vi "WS1050 36 DUT CV Curve Ver1.3.vi"() -> ()   [LabVIEW 2012]
uses:
  WS_VCAP Driver 029/Source/WSVCAP Shell/Type Defs/WSVCAP SHL I2C DUT Mask Mode Enum.ctl
panel:
  out "date string":string="5/19/2014"
  in  "Tab Control":T1(tab)
  in  "Sweep CP":bool=TRUE
  in  "Board#":string="BRD5"
  in  "Serial Number":string[][](table)=[["DUT", "SN"], ["DUT1", "1"], ["DUT2", "2"], ["DUT3", "3"], ["DUT4", "4"], ["DUT5", "5"], ["DUT6", "6"], ["DUT7", "7"], ["DUT8", "8"], ["DUT9", "9"], ["DUT10", "10"], ["DUT11", "11"], ["DUT12", "12"], ["DUT13", "13"], ["DUT14", "14"], ["DUT15", "15"], ["DUT16", "16"], ["DUT17", "17"], ["DUT18", "18"], ["DUT19", "19"], ["DUT20", "20"], ["DUT21", "21"], ["DUT22", "22"], ["DUT23", "23"], ["DUT24", "24"], ["DUT25", "25"], ["DUT26", "26"], ["DUT27", "27"], ["DUT28", "28"], ["DUT29", "29"], ["DUT30", "30"], ["DUT31", "31"], ["DUT32", "32"], ["DUT33", "33"], ["DUT34", "34"], ["DUT35", "35"], ["DUT36", "36"]]
  in  "Wafer#":string="T7-EB"
  in  "File Name":string="CP Sweep_WS1050_T7_EB_25C_BRD4_160706_1"
  in  "TMN DC\\CAP Data Log File Path":path=path "C:/WS1050 36 DUT Data"
  in  "Test Program":string="WS1050 36 DUT CV Curve Ver1.3"
  out "Current Date":string="8/28/2014"
  out "Current Time":string="0950"
  in  "Start Date":string="10/21/2014"
  in  "Start Time":string="1542"
  in  "Comment":string="CP Sweep RT"
  in  "OK Button":bool
  in  "Calibration":bool
  in  "Verify CP":bool
  in  "CP Setting":i32(ring) items=["CP OFF", "CP ON", "CP 35V", "CP 40V", "DVA ON", "DVA OFF", "REG1 ON", "REG1 OFF", "REG2 ON", "REG2 OFF", "REG3 ON", "REG3 OFF"]
  in  "Set VDD":dbl=3.3 format="%.3g"
  in  "Clock Rate (Hz)":dbl=1000000.0 caption="Meas Speed" format="%.1p Hz"
  out "AR  Measurent(Hz)":dbl
  in  "PS1 Source":refnum<visa-resource-name>="GPIB0::5::INSTR"
  in  "Ke2000":refnum<visa-resource-name>="GPIB0::9::INSTR"
  out "Simulate FPGA":bool
  out "Online":bool
  in  "Ke2400":refnum<visa-resource-name>="GPIB0::3::INSTR"
  in  "Initialize AD7747":bool
  in  "DUT Mask Mode":T2=enum."All"
  in  "RFFE Slave Address":u8=7 caption="Slave Address" format="0x%02x"
  out "Activity Log":string="05/19/2014 -- 12:24:35.853::WSVCAP::APP::Application Started\n05/19/2014 -- 12:24:37.606::WSVCAP::WSVCAP SHL::WR I2C-REG:0x0A;MASK:0xFFFFFFFFFFFF;C1 DATA:22:22:22:22:22:22:22:22:22:22:22:22:22:22:22:22;C2 DATA:22:22:22:22:22:22:22:22:22:22:22:22:22:22:22:22;C3 DATA:22:22:22:22:22:22:22:22:22:22:22:22:22:22:22:22\r\n05/19/2014 -- 12:24:37.773::WSVCAP::WSVCAP SHL::WR I2C-ST:0,0,4,1\r\n05/19/2014 -- 12:24:37.903::WSVCAP::WSVCAP SHL::RD I2C-BYTES:4;ADD:0x00;MASK:0xFFFFFFFFFFFF\r\n05/19/2014 -- 12:24:38.045::WSVCAP::WSVCAP SHL::RD I2C:C1 DATA:2:2:2:2:2:2:2:2:2:2:2:2:2:2:2:2|A7:A9:AA:82:82:7F:82:81:82:81:83:82:81:82:82:81|46:36:BB:88:44:A3:E9:2B:32:20:ED:25:BB:3D:68:B|2C:6A:EB:A7:22:56:FE:CC:36:82:D7:B0:3B:48:F9:CC;C2 DATA:2:2:2:2:2:2:2:2:2:2:2:2:2:2:2:2|94:94:94:80:80:80:80:80:81:7E:7E:81:80:7E:80:80|47:33:15:82:62:B:E8:1C:D7:C3:7D:41:7C:B7:4C:2A|C4:B4:AE:8:1E:D1:4E:37:11:C0:6F:63:42:9D:63:B5;C3 DATA:2:2:2:2:2:2:2:2:2:2:2:2:2:2:2:2|95:95:95:81:81:7E:81:80:84:7D:80:83:81:7E:7F:80|AB:C4:14:B5:7B:52:DF:C9:79:5D:5F:30:99:31:1E:F4|6E:5C:F7:A8:C3:EB:7B:EF:33:92:89:77:4D:67:75:DD;STATUS:0:0:4:0\r\n05/19/2014 -- 12:24:38.046::WSVCAP::WSVCAP SHL::WR I2C-REG:0x0A;MASK:0xFFFFFFFFFFFF;C1 DATA:22:22:22:22:22:22:22:22:22:22:22:22:22:22:22:22;C2 DATA:22:22:22:22:22:22:22:22:22:22:22:22:22:22:22:22;C3 DATA:22:22:22:22:22:22:22:22:22:22:22:22:22:22:22:22\r\n05/19/2014 -- 12:24:38.089::WSVCAP::WSVCAP SHL::WR I2C-ST:0,0,4,1\r\n05/19/2014 -- 12:24:38.219::WSVCAP::WSVCAP SHL::RD I2C-BYTES:4;ADD:0x00;MASK:0xFFFFFFFFFFFF\r\n05/19/2014 -- 12:24:38.362::WSVCAP::WSVCAP SHL::RD I2C:C1 DATA:2:2:2:2:2:2:2:2:2:2:2:2:2:2:2:2|A7:AB:AA:82:82:82:83:83:82:82:82:82:7F:82:82:81|4B:32:96:83:3E:61:43:17:25:62:AB:4D:A2:40:2E:5|3C:76:2B:B4:EE:E4:A9:1A:AA:A:26:C7:21:2E:87:5B;C2 DATA:2:2:2:2:2:2:2:2:2:2:2:2:2:2:2:2|94:94:94:80:80:80:80:80:80:7F:80:81:80:80:7F:80|4A:32:19:7D:19:6C:79:46:61:7F:4B:B8:A5:30:F3:14|B4:70:A:8C:9C:DC:43:FA:1E:A:C6:21:A:A9:13:F3;C3 DATA:2:2:2:2:2:2:2:2:2:2:2:2:2:2:2:2|95:97:94:81:80:81:82:81:80:7E:81:84:7F:81:80:80|B2:32:D0:A7:9E:4C:AB:D4:EE:D9:F0:82:B7:91:7:FF|C1:91:B6:3D:D8:E:1B:4F:9F:6A:F1:6C:E7:3F:7:BA;STATUS:0:0:4:0\r\n05/19/2014 -- 12:24:38.364::WSVCAP::WSVCAP SHL::WR I2C-REG:0x0A;MASK:0xFFFFFFFFFFFF;C1 DATA:22:22:22:22:22:22:22:22:22:22:22:22:22:22:22:22;C2 DATA:22:22:22:22:22:22:22:22:22:22:22:22:22:22:22:22;C3 DATA:22:22:22:22:22:22:22:22:22:22:22:22:22:22:22:22\r\n05/19/2014 -- 12:24:38.406::WSVCAP::WSVCAP SHL::WR I2C-ST:0,0,4,1\r\n05/19/2014 -- 12:24:38.536::WSVCAP::WSVCAP SHL::RD I2C-BYTES:4;ADD:0x00;MASK:0xFFFFFFFFFFFF\r\n05/19/2014 -- 12:24:38.678::WSVCAP::WSVCAP SHL::RD I2C:C1 DATA:2:2:2:2:2:2:2:2:2:2:2:2:2:2:2:2|A7:A9:AB:82:82:81:82:82:82:82:82:82:82:82:82:81|46:71:4C:87:43:3D:7F:FC:25:4F:8E:54:97:3E:60:8C|AA:F4:1F:B5:CE:43:1F:36:9:87:9C:78:86:5:B6:8E;C2 DATA:2:2:2:2:2:2:2:2:2:2:2:2:2:2:2:2|94:94:94:80:7F:7F:80:80:80:80:80:81:80:80:80:80|49:36:18:7D:6E:C5:E4:3C:81:2E:41:D3:75:71:E3:72|E8:D3:E6:D1:E0:48:AE:D4:54:D:E8:8E:B4:41:68:4;C3 DATA:2:2:2:2:2:2:2:2:2:2:2:2:2:2:2:2|95:95:95:81:7F:7F:81:81:81:81:81:84:81:81:82:81|B3:F5:90:AB:82:69:7B:93:D0:77:E8:D5:E8:8C:84:E8|B9:AC:EE:2B:B6:71:8F:4A:74:31:56:BB:8A:B7:A0:C8;STATUS:0:0:4:0\r\n05/19/2014 -- 12:24:38.681::WSVCAP::WSVCAP SHL::WR I2C-REG:0x0A;MASK:0xFFFFFFFFFFFF;C1 DATA:22:22:22:22:22:22:22:22:22:22:22:22:22:22:22:22;C2 DATA:22:22:22:22:22:22:22:22:22:22:22:22:22:22:22:22;C3 DATA:22:22:22:22:22:22:22:22:22:22:22:22:22:22:22:22\r\n05/19/2014 -- 12:24:38.723::WSVCAP::WSVCAP SHL::WR I2C-ST:0,0,4,1\r\n05/19/2014 -- 12:24:38.854::WSVCAP::WSVCAP SHL::RD I2C-BYTES:4;ADD:0x00;MASK:0xFFFFFFFFFFFF\r\n05/19/2014 -- 12:24:38.996::WSVCAP::WSVCAP SHL::RD I2C:C1 DATA:2:2:2:2:2:2:2:2:2:2:2:2:2:2:2:2|A7:A9:AA:82:82:7F:83:81:82:81:84:82:7F:82:7F:82|43:FB:E:7F:3C:AD:35:35:26:A2:6C:21:4B:3D:8:6|63:9A:E1:F3:95:32:91:42:90:3C:78:1F:5C:D7:5F:D8;C2 DATA:2:2:2:2:2:2:2:2:2:2:2:2:2:2:2:2|94:94:94:80:80:80:80:80:81:80:7E:81:80:7E:7F:80|48:36:18:7F:5E:3D:69:83:DE:AE:A1:9E:31:AE:BB:96|15:A0:44:17:13:FD:CC:C8:6D:B2:EF:A7:C:C7:3B:F;C3 DATA:2:2:2:2:2:2:2:2:2:2:2:2:2:2:2:2|95:96:94:81:81:7E:82:80:84:80:80:84:7F:7E:7D:82|AD:3B:6D:A9:7C:57:9D:F5:7A:96:23:5C:36:2D:ED:5A|CD:46:DB:3B:C7:BD:70:60:33:B8:B:F7:63:A:51:4D;STATUS:0:0:4:0\r\n05/19/2014 -- 12:24:38.998::WSVCAP::WSVCAP SHL::WR I2C-REG:0x0A;MASK:0xFFFFFFFFFFFF;C1 DATA:22:22:22:22:22:22:22:22:22:22:22:22:22:22:22:22;C2 DATA:22:22:22:22:22:22:22:22:22:22:22:22:22:22:22:22;C3 DATA:22:22:22:22:22:22:22:22:22:22:22:22:22:22:22:22\r\n05/19/2014 -- 12:24:39.040::WSVCAP::WSVCAP SHL::WR I2C-ST:0,0,4,1\r\n05/19/2014 -- 12:24:39.170::WSVCAP::WSVCAP SHL::RD I2C-BYTES:4;ADD:0x00;MASK:0xFFFFFFFFFFFF\r\n05/19/2014 -- 12:24:39.311::WSVCAP::WSVCAP SHL::RD I2C:C1 DATA:2:2:2:2:2:2:2:2:2:2:2:2:2:2:2:2|A7:AA:AB:82:82:81:82:81:82:81:82:82:82:82:7F:82|44:F1:90:87:45:44:C8:2C:2C:F1:FC:1B:94:3B:3C:75|4A:49:95:19:99:73:64:3:23:24:F3:A2:5E:7F:C4:B6;C2 DATA:2:2:2:2:2:2:2:2:2:2:2:2:2:2:2:2|94:94:94:80:80:80:80:7F:80:80:7E:80:80:7E:7F:80|4C:36:17:7D:A8:9F:DE:C7:53:6D:8A:F4:41:A5:C6:E0|90:2E:24:C:D9:22:E4:76:3B:40:1D:53:33:B1:3E:4D;C3 DATA:2:2:2:2:2:2:2:2:2:2:2:2:2:2:2:2|95:97:95:81:81:7F:81:80:80:81:7F:82:81:7E:7D:82|AE:2B:A7:AB:CC:CD:A4:38:FD:17:80:F2:92:2D:45:C4|76:E5:D:B9:AD:B5:BA:8D:28:32:9E:42:B7:20:4A:D9;STATUS:0:0:4:0\r\n05/19/2014 -- 12:24:39.313::WSVCAP::WSVCAP SHL::WR I2C-REG:0x0A;MASK:0xFFFFFFFFFFFF;C1 DATA:22:22:22:22:22:22:22:22:22:22:22:22:22:22:22:22;C2 DATA:22:22:22:22:22:22:22:22:22:22:22:22:22:22:22:22;C3 DATA:22:22:22:22:22:22:22:22:22:22:22:22:22:22:22:22\r\n05/19/2014 -- 12:24:39.355::WSVCAP::WSVCAP SHL::WR I2C-ST:0,0,4,1\r\n05/19/2014 -- 12:24:39.486::WSVCAP::WSVCAP SHL::RD I2C-BYTES:4;ADD:0x00;MASK:0xFFFFFFFFFFFF\r\n05/19/2014 -- 12:24:39.628::WSVCAP::WSVCAP SHL::RD I2C:C1 DATA:2:2:2:2:2:2:2:2:2:2:2:2:2:2:2:2|A7:A9:AA:82:82:82:83:82:82:82:82:82:7F:82:7F:82|47:18:E4:87:3E:E7:6:65:25:92:37:38:A8:3E:89:85|7C:A7:7:2B:A3:7A:EC:EF:89:ED:F4:D3:D8:BC:3A:F5;C2 DATA:2:2:2:2:2:2:2:2:2:2:2:2:2:2:2:2|94:94:94:80:7F:80:80:7F:81:80:7E:80:80:80:81:80|49:37:17:80:76:25:6A:F8:DF:55:97:4D:B8:5B:2B:B1|13:E3:9A:3E:1A:2D:4F:B6:DB:E9:61:FA:8B:D6:9:CC;C3 DATA:2:2:2:2:2:2:2:2:2:2:2:2:2:2:2:2|95:95:95:81:7F:80:82:81:84:80:7F:81:80:81:7F:82|AF:93:3B:AF:5B:11:82:E4:7E:C3:2D:72:9:96:D9:A|DB:96:F2:10:5F:64:9A:C6:98:12:27:7D:10:D3:20:D9;STATUS:0:0:4:0\r\n05/19/2014 -- 12:24:40.132::WSVCAP::WSVCAP SHL::CLOSE\r\n"
  out "IDD Brd(uA)":string
  in  "Control Panel":T3={"E-CAL"=FALSE, "DVA"=FALSE, "CP Sweep"=TRUE}
  out "E-CAL":bool
  out "DVA":bool
  out "CP Sweep":bool
  in  "Lot#":string="WS1050"
  out "AD7747 Values":string[][](table)
  in  "Freq(Hz)":string="NA"
  in  "WS1050/51":bool=TRUE
  in  "Serialize":bool
  in  "Start No":i32=1
  in  "VPI Name":string[](array[string])=["All Drivers ON"]
  in  "VPI_Cmd":string[](array[string])=["3B"]
  in  "Temperature":string="25C"
  in  "Command":string[](array[string])=["0702013B3B3B", "070201000000", "0702013B0000"]
  in  "Cycle (X1000)":dbl=2.0
  in  "Post CMd Delay":dbl[](array[numeric])=[1.2e-05, 5.4e-05, 1.8e-05] min=0.0 max=0.5 format="%#.0p s"
  in  "Init Cycle":bool=TRUE
  out "Cycle Count":u64 min=1 max=4 step=1
  in  "C3 Cap DAC":u8=128 caption="B Data In" format="0x%02x"
  in  "C2 Cap DAC":u8=128 caption="B Data In" format="0x%02x"
  in  "C1 Cap DAC":u8=128 caption="B Data In" format="0x%02x"
  out "NOM IDD OFF(uA)":string
  out "Previous Time":string="12:20:26 PM"
  out "STATUS":string="Idle...."
  out "RB Reg for HD/Cycle":string[](array[string])
  out "VPI C2":string[][](table)
  out "VPI C3":string[][](table)
  out "NOM IDD ON (uA)":string
  in  "stop":bool
  out "IDD Stdby(uA)":string="2.606990E+0"
  out "VPI C1":string[][](table)
  out "Loop Completed":i32
  in  "error in (no error)":errorcluster
  out "error out":errorcluster
  in  "Bank 2":i32(ring)=1 items=["C1", "C2", "C3", "D_C1", "D_C2", "D_C3"]
  out "DeltaC Change_1":dbl[][](graph) caption="(Y) Multi Plot 2"
  out "DeltaC Change_2":dbl[][](graph) caption="(Y) Multi Plot 2"
  out "DeltaC Change_3":dbl[][](graph) caption="(Y) Multi Plot 2"
  in  "Debug":bool
  in  "No of Rows\nFrom Spread Sheet":i32
  in  "Plot Delta Cmin":bool=TRUE
  in  "Plot":T4(ring)
  in  "Bank 1":i32(ring) items=["C1", "C2", "C3", "D_C1", "D_C2", "D_C3"]
  in  "Bank 3":i32(ring)=2 items=["C1", "C2", "C3", "D_C1", "D_C2", "D_C3"]
  in  "Col C1":i32=5
  in  "Col C2":i32=6
  in  "Col C3":i32=7
  # "Company:  WiSpry Inc\n20 Fairbanks Ste 198 Irvine CA 92618\n\nAuthor:  Andy V Tran\nCreated:  07/07/2016\nLabVIEW 2012 Pro\nTest Program:  WS1050 36 DUT \nCP Sweep ver1.3\nFPGA: WS_VCAP Driver 029"
  # "Note for CP CV Sweep:\n\n1.  CP will sweep as follow:\n     a.  Low to High, from 23.75V to 55V, step 0.75V\n     b.  Low to High to Low, from 23.75V to 55V to 23.75V, step 0.75V\n\n2.  CP sweep by banks, C1, C2 then C3"
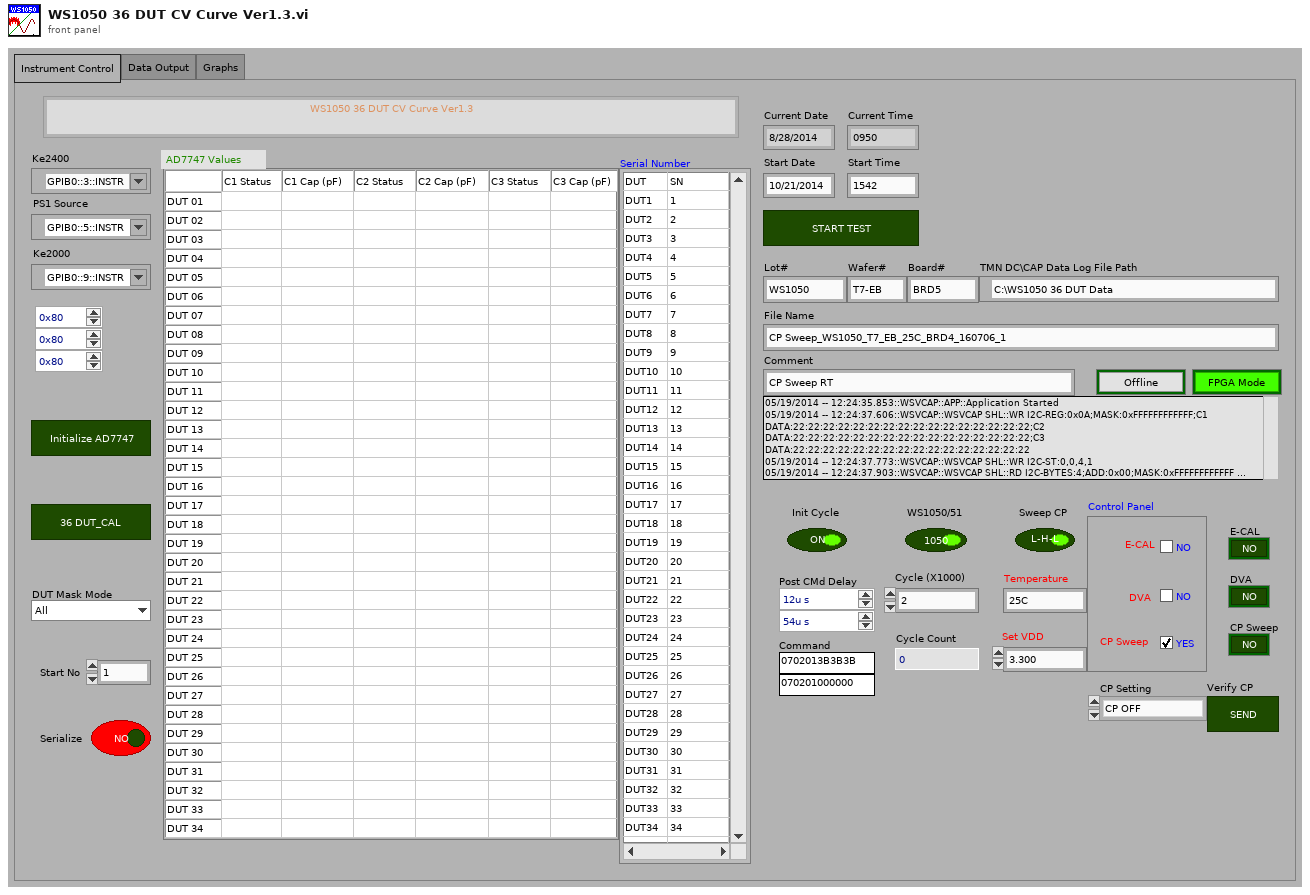
[diagram p1: front panel]
types:
  T1 = enum32{"Instrument Control", "Data Output", "Graphs"}
  T2 = typedef "WSVCAP SHL I2C DUT Mask Mode Enum.ctl" = enum16{"Custom", "C1", "C2", "C3", "All"}
  T3 = cluster{"E-CAL":bool, "DVA":bool, "CP Sweep":bool}
  T4 = enum16{"ALL DUTs", "DUT 01", "DUT 02", "DUT 03", "DUT 04", "DUT 05", "DUT 06", "DUT 07", "DUT 08", "DUT 09", "DUT 10", "DUT 11", "DUT 12", "DUT 13", "DUT 14", "DUT 15", "DUT 16", "DUT 17", "DUT 18", "DUT 19", "DUT 20", "DUT 21", "DUT 22", "DUT 23", "DUT 24", "DUT 25", "DUT 26", "DUT 27", "DUT 28", "DUT 29", "DUT 30", "DUT 31", "DUT 32", "DUT 33", "DUT 34", "DUT 35", "DUT 36"}
  T5 = typedef "WSVCAP SHL Core System Cluster.ctl" = cluster{"Settings":T6, "FPGA Resource":tag, "Online":bool, "I2C Wait Ticks":u32, "SPI Wait Ticks":u32, "RFFE Wait Ticks":u32}
  T6 = typedef "WSVCAP SHL I2C Settings Cluster.ctl" = cluster{"FPGA Resource Name":string, "I2C Slave Address":u8, "I2C Clock Rate (Hz)":dbl, "SPI Clock Rate (Hz)":dbl, "RFFE Slave Address":u8, "RFFE Clock Rate (Hz)":dbl, "Simulate FPGA":bool, "C1 Cap DAC Default":u8, "C2 Cap DAC Default":u8, "C3 Cap DAC Default":u8}
  T7 = enum16{"Idle...", "Voltage 1", "Voltage 2", "Voltage 3"}
  T8 = enum16{"Idle...", "Voltage 1", "Voltage 2", "Voltage 3"}[]
  T9 = cluster{"Test Program ":string, "Comment":string, "Data Out":string, "Data Out":string, string, string, "Data Out":string, "Data Out":string, "string":string, "Freq(Hz)":string, "Board#":string}
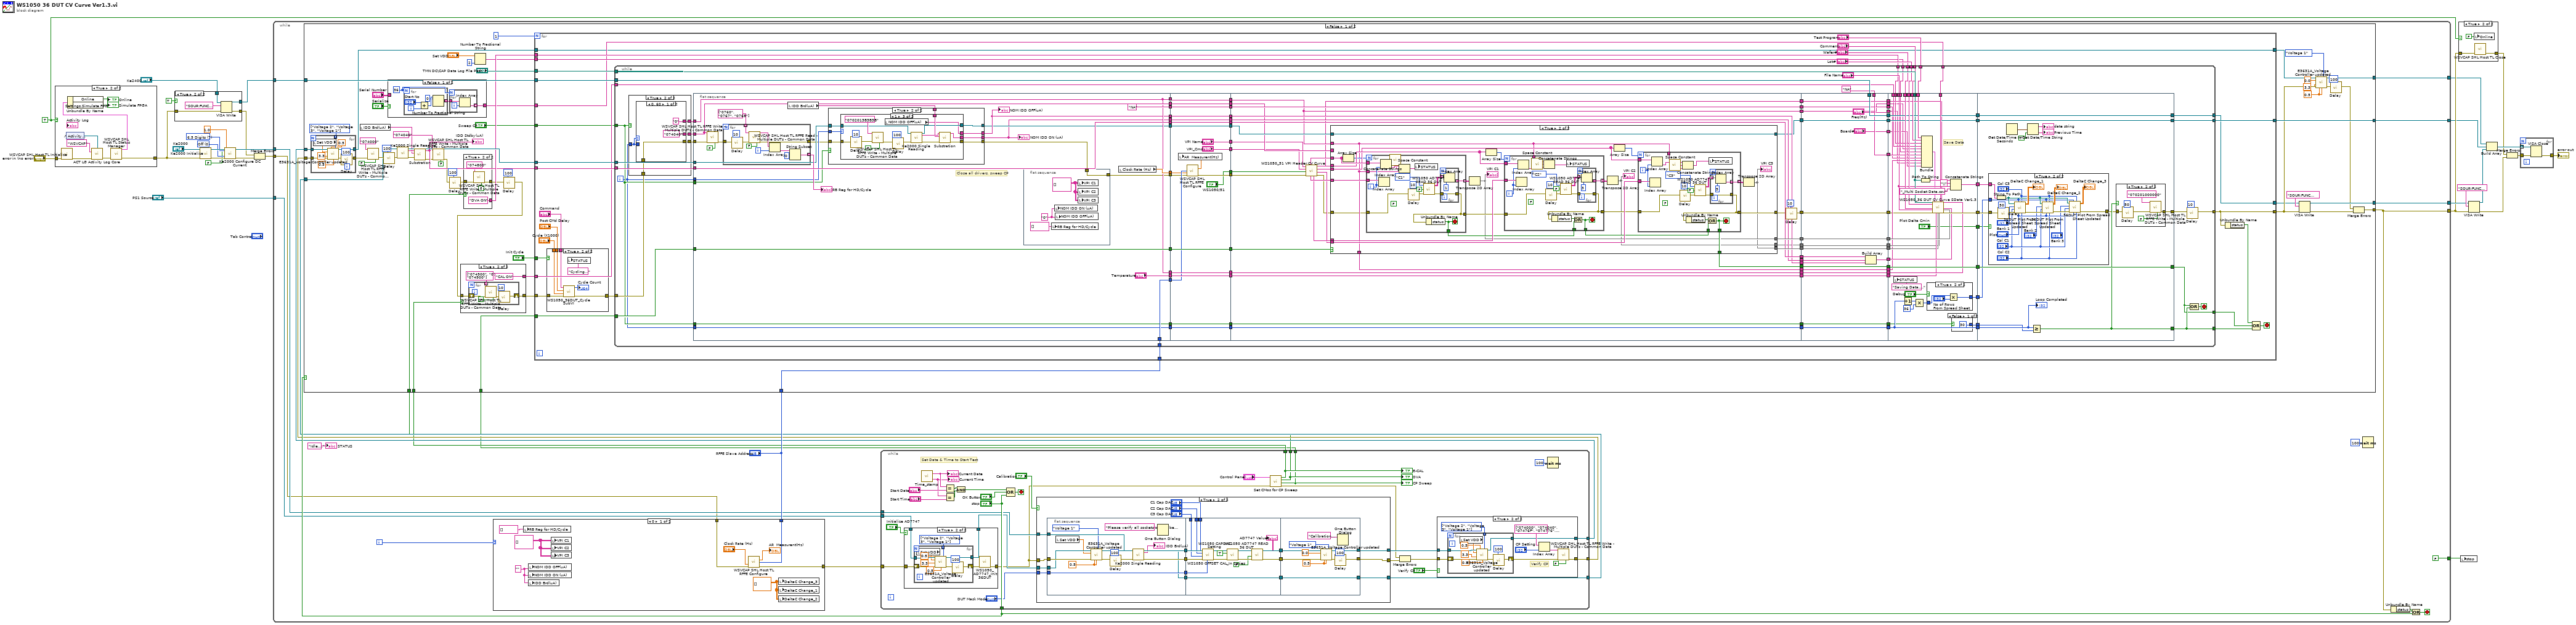
[diagram p0: block diagram]
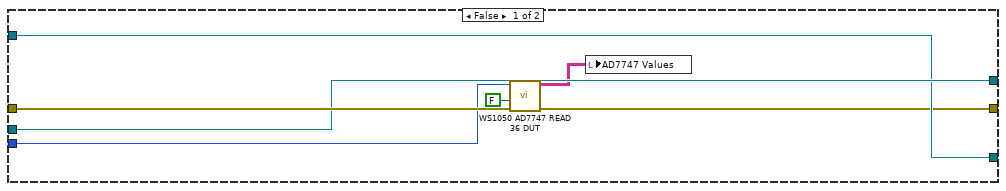
[diagram p8: hidden frame]
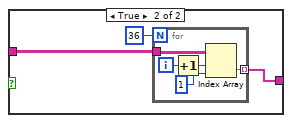
[diagram p9: hidden frame]
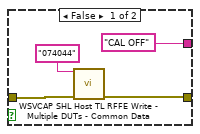
[diagram p10: hidden frame]
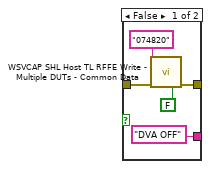
[diagram p11: hidden frame]
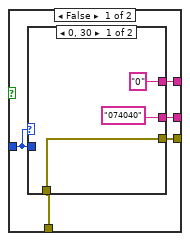
[diagram p13: hidden frame]
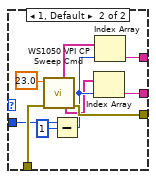
[diagram p14: hidden frame]
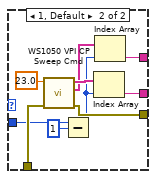
[diagram p15: hidden frame]
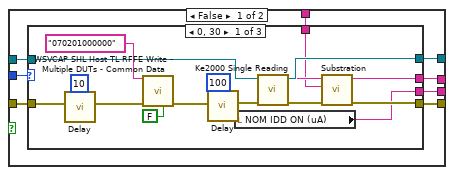
[diagram p16: hidden frame]
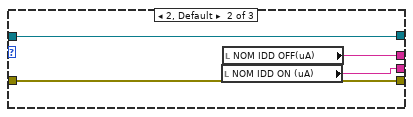
[diagram p17: hidden frame]
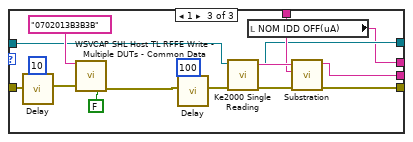
[diagram p18: hidden frame]
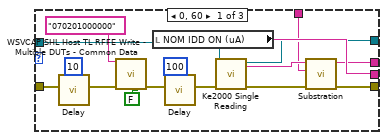
[diagram p19: hidden frame]
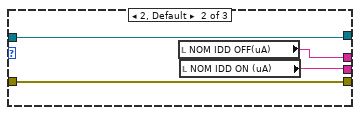
[diagram p20: hidden frame]
diagram:
  w22 = TRUE
  w26 = u16 0 items=["Off", "Moving Filter", "Repeating Filter"] ("Digital Filter (0: Off)")
  w27 = u16 7 items=["3.5 Digits"=4, "4.5 Digits"=5, "5.5 Digits"=6, "6.5 Digits"=7] ("Resolution (7: 6.5 digits)")
  n1 = case shown="True" w22 {
    tunnel: "error in (no error)" -> [w31 w32]
    tunnel: [w31 w39] -> w12
    frame False {
    }
    frame True {
      n2 = call "WSVCAP SHL Host TL Initialize.vi"("error in"=w32) -> ("error out"=w33:errorcluster)  [unwired: 13 in, 1 out]
      n3 = control-ref of="Activity Log"() -> (w35:refnum<vi>)
      n4 = call "ACT LG Activity Log Core.vi"("Display Ref"=w35, "Source"="WSVCAP", "Error In (no error)"=w33) -> ("Error Out"=w34:errorcluster)  [unwired: 11 in, 1 out]
      n5 = call "WSVCAP SHL Host TL Status Manager.vi"("error in"=w34) -> ("System Out"=w40:T5, "error out"=w39:errorcluster)  [unwired: 13 in]
      n6 = Unbundle By Name(w40) -> ("Online"=→"Online":bool, "Settings.Simulate FPGA"=→"Simulate FPGA":bool)
    }
  }
  n7 = case shown="True" TRUE {
    tunnel: w12 -> [w41 w46]
    tunnel: [w42 w45] -> w19
    tunnel: [w41 w44] -> w15
    tunnel: "Ke2400" -> [w42 w43]
    frame False {
    }
    frame True {
      n8 = VISA Write(VISA resource name=w43, write buffer="SOUR:FUNC VOLT;VOLT:MODE FIX;RANG 100;LEV 0.0;:SENS:FUNC \"CURR\";CURR:PROT 60E-3;RANG 100E-3;:OUTP ON", error in (no error)=w46) -> (VISA resource name out=w45:refnum<visa-resource-name>, error out=w44:errorcluster)  [unwired: 1 out]
    }
  }
  n9 = call "Ke2000 Initialize.vi"("error in (no error)"=w12, "VISA resource name"="Ke2000") -> ("error out"=w28:errorcluster, "VISA resource name out"=w29:refnum<visa-resource-name>)  [unwired: 8 in]
  n10 = call "Ke2000 Configure DC Current.vi"("Resolution (7: 6.5 digits)"=w27, "Digital Filter (0: Off)"=w26, "Auto Range? (T: Auto)"=FALSE, "error in"=w28, "Custom Range (0 A)"=1.0, "VISA resource name"=w29) -> ("error out"=w13:errorcluster, "VISA resource name out"=w24:refnum<visa-resource-name>)  [unwired: 4 in]
  n11 = Merge Errors(w15, w13) -> (w20:errorcluster)
  n12 = while {
    tunnel: w20 -> [w53]
    tunnel: [w54] -> w16
    tunnel: "PS1 Source" -> [w58]
    tunnel: w24 -> [w59]
    tunnel: [w67] -> w8
    tunnel: [w66] -> w9
    tunnel: w19 -> [w64]
    tunnel: [w63] -> w17
    tunnel: [FALSE ("stop")] -> w10
    i -> [w65]
    stop <- w69 stop-if-true
    n13 = case shown="0" w65 {
      tunnel: w53 -> [w79 w80]
      tunnel: [w78 w80] -> w61
      tunnel: "RFFE Slave Address" -> [w76 _]
      frame 0 {
        w72 = dbl[][] []
        w71 = "" ("uA")
        w73 = string[][] []
        n14 = local write "RB Reg for HD/Cycle"(string[] [] ("EFuse Read back")) -> ()
        n15 = local write "NOM IDD OFF(uA)"(w71) -> ()
        n16 = local write "NOM IDD ON (uA)"(w71) -> ()
        n17 = local write "IDD Brd(uA)"(w71) -> ()
        n18 = local write "VPI C1"(w73) -> ()
        n19 = local write "VPI C2"(w73) -> ()
        n20 = local write "VPI C3"(w73) -> ()
        n21 = call "WSVCAP SHL Host TL RFFE Configure.vi"("RFFE Slave Address"=w76, "Clock Rate (Hz)"="Clock Rate (Hz)", "error in"=w79) -> ("Actual Rate (Hz)"=→"AR  Measurent(Hz)":dbl, "error out"=w78:errorcluster)  [unwired: 11 in]
        n22 = local write "DeltaC Change_3"(w72) -> ()
        n23 = local write "DeltaC Change_1"(w72) -> ()
        n24 = local write "DeltaC Change_2"(w72) -> ()
      }
      frame 1, Default {
      }
    }
    n25 = while {
      tunnel: ["stop"] -> w62
      tunnel: w61 -> [w97]
      tunnel: [w89] -> w55
      tunnel: w58 -> [w96]
      tunnel: w59 -> [w91]
      tunnel: [w92] -> w57
      tunnel: [w90] -> w56
      tunnel: [w88] -> w52
      tunnel: [w87] -> w51
      tunnel: [w86] -> w50
      stop <- w104 stop-if-true
      # "Set Date & Time to Start Test"
      n26 = case shown="True" "Initialize AD7747" {
        tunnel: w97 -> [w113 w118]
        tunnel: [w113 w114] -> w85
        tunnel: w96 -> [w112 w116]
        tunnel: [w112 w115] -> w95
        frame False {
        }
        frame True {
          w119 = T8 [enum."Voltage 2", enum."Voltage 3", enum."Voltage 1"] items=["Idle...", "Voltage 1", "Voltage 2", "Voltage 3"]
          n27 = for {
            tunnel: w116 -> [w129]
            tunnel: w119 -> [w127] mode=indexing
            tunnel: [w126] -> w115
            shift-right: [w122] -> w117
            shift-left: w118 -> [w130]
            n28 = local read "Set VDD"() -> (w125:dbl)
            n29 = call "E3631A_Voltage Controller updated.vi"("VISA resource name"=w129, "I_VDD(A)"=0.5, "Channel Controller"=w127, "Voltage 1"=w125, "Voltage 2"=3.3, "error in (no error)"=w130, "I_3.3V (A)"=0.5) -> ("VISA resource name out"=w126:refnum<visa-resource-name>, "error out"=w121:errorcluster)  [unwired: 7 in]
            n30 = call "Delay.vi"("milliseconds to wait"=u32 100, "error in (no error)"=w121) -> ("error out"=w122:errorcluster)  [unwired: 9 in]
          }
          n31 = call "WS1050_AD7747_Init 36DUT.vi"("error in"=w117) -> ("error out"=w114:errorcluster)  [unwired: 10 in]
        }
      }
      n32 = call "Time_stamp.vi"() -> ("date/time string"=w109:string, "date string"=w111:string)  [unwired: 2 in]
      "Current Date" <- w111
      "Current Time" <- w109
      n33 = Equal?(x=w111, y="Start Date") -> (x = y?=w107:bool)
      n34 = Equal?(x=w109, y="Start Time") -> (x = y?=w106:bool)
      n35 = And(x=w107, y=w106) -> (x .and. y?=w103:bool)
      n36 = Compound Arithmetic op=OR(w103, "OK Button", "stop") -> (w104:bool)
      n37 = case shown="True" "Calibration" {
        tunnel: w85 -> [w160 w177]
        tunnel: [w154 w174] -> w83
        tunnel: w95 -> [w159 w173]
        tunnel: "DUT Mask Mode" -> [w158 w169]
        tunnel: [w159 w168] -> w93
        tunnel: w91 -> [w157 w164]
        tunnel: [w157 w161] -> w90
        frame False {
          n38 = call "WS1050 AD7747 READ 36 DUT.vi"("error in"=w160, "Log (T)"=FALSE, "DUT Mask Mode (All)"=w158) -> ("error out"=w154:errorcluster, "AD7747 Values"=w155:string[][])  [unwired: 7 in]
          n39 = local write "AD7747 Values"(w155) -> ()
        }
        frame True {
          n40 = flat-sequence {
            tunnel: w177 -> [w191]
            tunnel: [w186] -> w176
            tunnel: w173 -> [w190]
            tunnel: [w189] -> w172
            tunnel: w169 -> [w188]
            tunnel: [w188] -> w170
            tunnel: w164 -> [w184]
            tunnel: [w183] -> w163
            tunnel: w176 -> [w205]
            tunnel: [w204] -> w175
            tunnel: w172 -> [w203]
            tunnel: [w203] -> w171
            tunnel: w170 -> [w202]
            tunnel: "C1 Cap DAC" -> [w198]
            tunnel: "C2 Cap DAC" -> [w197]
            tunnel: "C3 Cap DAC" -> [w196]
            tunnel: w163 -> [w195]
            tunnel: [w195] -> w162
            tunnel: w175 -> [w213]
            tunnel: [w215] -> w174
            tunnel: w171 -> [w214]
            tunnel: [w212] -> w168
            tunnel: w162 -> [w211]
            tunnel: [w211] -> w161
            frame #0 {
              w178 = 0.5 ("I_VDD(A)")
              n41 = local read "Set VDD"() -> (w180:dbl)
              n42 = call "E3631A_Voltage Controller updated.vi"("VISA resource name"=w190, "I_VDD(A)"=w178, "Channel Controller"=T7."Voltage 1", "Voltage 1"=w180, "error in (no error)"=w191, "I_3.3V (A)"=w178) -> ("VISA resource name out"=w189:refnum<visa-resource-name>, "error out"=w181:errorcluster)  [unwired: 8 in]
              n43 = call "Delay.vi"("milliseconds to wait"=u32 100, "error in (no error)"=w181) -> ("error out"=w185:errorcluster)  [unwired: 9 in]
              n44 = call "Ke2000 Single Reading.vi"("error in (no error)"=w185, "VISA resource name"=w184) -> ("error out"=w186:errorcluster, "VISA resource name out"=w183:refnum<visa-resource-name>, "uA"=→"IDD Brd(uA)":string)  [unwired: 5 in, 2 out]
              n45 = One Button Dialog(message="Please verify all sockets should be empty...") -> ()  [unwired: 1 in, 1 out]
            }
            frame #1 {
              n46 = call "WS1050 CAPDAC Setting.vi"("DUT Mask Mode (All)"=w202, "error in"=w205, "C3 Cap DAC"=w196, "C2 Cap DAC"=w197, "C1 Cap DAC"=w198) -> ("error out"=w200:errorcluster)  [unwired: 6 in]
              n47 = call "WS1050 OFFSET CAL_In Series.vi"("error in"=w200, "OFFSET CAL"=TRUE ("Read?")) -> ("error out"=w199:errorcluster)  [unwired: 9 in]
              n48 = call "WS1050 AD7747 READ 36 DUT.vi"("error in"=w199, "Log (T)"=FALSE, "DUT Mask Mode (All)"=w202) -> ("error out"=w204:errorcluster, "AD7747 Values"=→"AD7747 Values":string[][])  [unwired: 7 in]
            }
            frame #2 {
              w206 = 0.5 ("I_3.3V (A)")
              n49 = call "E3631A_Voltage Controller updated.vi"("VISA resource name"=w214, "I_VDD(A)"=w206, "Channel Controller"=T7."Voltage 1", "Voltage 1"=0.0, "error in (no error)"=w213, "I_3.3V (A)"=w206) -> ("VISA resource name out"=w212:refnum<visa-resource-name>, "error out"=w208:errorcluster)  [unwired: 8 in]
              n50 = call "Delay.vi"("milliseconds to wait"=u32 100, "error in (no error)"=w208) -> ("error out"=w215:errorcluster)  [unwired: 9 in]
              n51 = One Button Dialog(message="Calibration Completed....") -> ()  [unwired: 1 in, 1 out]
            }
          }
        }
      }
      n52 = call "Set CMos for CP Sweep.vi"("error in (no error)"=w85, "Control Panel"="Control Panel") -> ("error out"=w82:errorcluster, "CP Sweep"=w86:bool, "DVA"=w87:bool, "E-CAL"=w88:bool)  [unwired: 6 in]
      "E-CAL" <- w88
      "CP Sweep" <- w86
      "DVA" <- w87
      n53 = Merge Errors(w82, w83) -> (w84:errorcluster)
      n54 = case shown="True" "Verify CP" {
        tunnel: [w131 w135] -> w89
        tunnel: w93 -> [w132 w138]
        tunnel: [w132 w136] -> w92
        tunnel: w84 -> [w131 w134]
        frame False {
        }
        frame True {
          w139 = T8 [enum."Voltage 2", enum."Voltage 3", enum."Voltage 1"] items=["Idle...", "Voltage 1", "Voltage 2", "Voltage 3"]
          # "Verify CP"
          n55 = for {
            tunnel: w138 -> [w152]
            tunnel: w139 -> [w150] mode=indexing
            shift-right: [w147] -> w137
            shift-left: w134 -> [w153]
            tunnel: [w145] -> w136
            n56 = local read "Set VDD"() -> (w149:dbl)
            n57 = call "E3631A_Voltage Controller updated.vi"("VISA resource name"=w152, "I_VDD(A)"=0.5, "Channel Controller"=w150, "Voltage 1"=w149, "Voltage 2"=3.3, "error in (no error)"=w153, "I_3.3V (A)"=0.5) -> ("VISA resource name out"=w145:refnum<visa-resource-name>, "error out"=w148:errorcluster)  [unwired: 7 in]
            n58 = call "Delay.vi"("milliseconds to wait"=u32 100, "error in (no error)"=w148) -> ("error out"=w147:errorcluster)  [unwired: 9 in]
          }
          n59 = Index Array(array=string[] ["074000", "074040", "07476F", "074776", "074800", "074820", "07413B", "074100", "07423B", "074200", "07433B", "074300"], index="CP Setting") -> (element=w140:string)
          n60 = call "WSVCAP SHL Host TL RFFE Write - Multiple DUTs - Common Data.vi"("Data Out"=w140, "error in"=w137, "Log (T)"=FALSE) -> ("error out"=w135:errorcluster)  [unwired: 12 in]
        }
      }
      n61 = Wait (ms)(milliseconds to wait=u32 100 ("millisecond multiple")) -> ()  [unwired: 1 out]
    }
    n62 = case shown="False" w62 {
      tunnel: w55 -> [w275 w902]
      tunnel: [w262 w902] -> w54
      tunnel: w57 -> [w274 w900]
      tunnel: w56 -> [w267 w901]
      tunnel: [w272 w901] -> w67
      tunnel: [w271 w900] -> w66
      tunnel: w64 -> [w264 w899]
      tunnel: [w261 w899] -> w63
      tunnel: "RFFE Slave Address" -> [w259 _]
      tunnel: w52 -> [w238 _]
      tunnel: w51 -> [w221 _]
      tunnel: w50 -> [w237 _]
      frame False {
        w222 = 0.5 ("I_3.3V (A)")
        w273 = T8 [enum."Voltage 2", enum."Voltage 3", enum."Voltage 1"] items=["Idle...", "Voltage 1", "Voltage 2", "Voltage 3"]
        n63 = for {
          tunnel: w275 -> [w898]
          tunnel: w274 -> [w897]
          tunnel: w273 -> [w895] mode=indexing
          tunnel: [w890] -> w269
          tunnel: [w894] -> w260
          n64 = local read "Set VDD"() -> (w893:dbl)
          n65 = call "E3631A_Voltage Controller updated.vi"("VISA resource name"=w897, "I_VDD(A)"=0.5, "Channel Controller"=w895, "Voltage 1"=w893, "Voltage 2"=3.3, "error in (no error)"=w898, "I_3.3V (A)"=0.5) -> ("VISA resource name out"=w894:refnum<visa-resource-name>, "error out"=w891:errorcluster)  [unwired: 7 in]
          n66 = call "Delay.vi"("milliseconds to wait"=u32 100, "error in (no error)"=w891) -> ("error out"=w890:errorcluster)  [unwired: 9 in]
        }
        n67 = local read "IDD Brd(uA)"() -> (w248:string)
        n68 = call "WSVCAP SHL Host TL RFFE Write - Multiple DUTs - Common Data.vi"("Data Out"="074000", "error in"=w269, "Log (T)"=FALSE) -> ("error out"=w270:errorcluster)  [unwired: 12 in]
        n69 = call "Delay.vi"("milliseconds to wait"=u32 100, "error in (no error)"=w270) -> ("error out"=w268:errorcluster)  [unwired: 9 in]
        n70 = case shown="False" "Serialize" {
          tunnel: [w277 w288] -> w239
          tunnel: "Serial Number" -> [_ w287]
          frame False {
            w276 = 36
            n71 = for {
              N: w276 -> [_]
              tunnel: [w282] -> w278 mode=indexing
              i -> [w286]
              n72 = Add(x="Start No", y=w286) -> (x+y=w284:i32)
              n73 = Number To Fractional String(number=w284, precision (6)=i16 0) -> (F-format string=w282:string)  [unwired: 2 in]
            }
            n74 = for {
              N: w276 -> [_]
              tunnel: w278 -> [w281]
              tunnel: [w280] -> w277 mode=indexing
              i -> [w279]
              n75 = Index Array(array=w281, index=w279) -> (element=w280:string)
            }
          }
          frame True {
            n76 = for {
              N: 36 -> [_]
              tunnel: w287 -> [w294]
              tunnel: [w292] -> w288 mode=indexing
              i -> [w291]
              n77 = Increment(x=w291) -> (x+1=w290:i32)
              n78 = Index Array(array=w294, index (row)=w290, index (col)=1 ("disabled index (col)")) -> (element=w292:string)
            }
          }
        }
        n79 = call "Ke2000 Single Reading.vi"("error in (no error)"=w268, "VISA resource name"=w267) -> ("error out"=w249:errorcluster, "VISA resource name out"=w266:refnum<visa-resource-name>, "uA"=w251:string)  [unwired: 5 in, 2 out]
        n80 = call "Substration.vi"("error in (no error)"=w249, "Input2"=w248, "Input1"=w251) -> ("error out"=w233:errorcluster, "In1 - In2"=w250:string)  [unwired: 7 in]
        "IDD Stdby(uA)" <- w250
        n81 = call "WSVCAP SHL Host TL RFFE Write - Multiple DUTs - Common Data.vi"("Data Out"="074040", "error in"=w233, "Log (T)"=FALSE) -> ("error out"=w218:errorcluster)  [unwired: 12 in]
        n82 = call "Delay.vi"("milliseconds to wait"=u32 100, "error in (no error)"=w218) -> ("error out"=w257:errorcluster)  [unwired: 9 in]
        n83 = case shown="True" w221 {
          tunnel: w257 -> [w313 w316]
          tunnel: [w312 w314] -> w255
          tunnel: ["DVA OFF" ("Data Out") "DVA ON" ("Data Out")] -> w256
          frame False {
            n84 = call "WSVCAP SHL Host TL RFFE Write - Multiple DUTs - Common Data.vi"("Data Out"="074820", "error in"=w313, "Log (T)"=FALSE) -> ("error out"=w312:errorcluster)  [unwired: 12 in]
          }
          frame True {
            n85 = call "WSVCAP SHL Host TL RFFE Write - Multiple DUTs - Common Data.vi"("Data Out"="074800", "error in"=w316, "Log (T)"=FALSE) -> ("error out"=w314:errorcluster)  [unwired: 12 in]
          }
        }
        n86 = Number To Fractional String(number="Set VDD", precision (6)=i16 2) -> (F-format string=w253:string)  [unwired: 2 in]
        n87 = call "Delay.vi"("milliseconds to wait"=u32 100, "error in (no error)"=w255) -> ("error out"=w243:errorcluster)  [unwired: 9 in]
        n88 = case shown="True" w238 {
          tunnel: w243 -> [w298 w300]
          tunnel: [w295 w299] -> w242
          tunnel: ["CAL OFF" ("Data Out") "CAL ON" ("Data Out")] -> w244
          frame False {
            n89 = call "WSVCAP SHL Host TL RFFE Write - Multiple DUTs - Common Data.vi"("Data Out"="074044", "error in"=w298) -> ("error out"=w295:errorcluster)  [unwired: 13 in]
          }
          frame True {
            n90 = for {
              tunnel: string[] ["074900", "074920", "074900"] -> [w308] mode=indexing
              shift-right: [w304] -> w299
              shift-left: w300 -> [w305]
              n91 = call "WSVCAP SHL Host TL RFFE Write - Multiple DUTs - Common Data.vi"("Data Out"=w308, "error in"=w305, "Log (T)"=FALSE) -> ("error out"=w307:errorcluster)  [unwired: 12 in]
              n92 = call "Delay.vi"("milliseconds to wait"=u32 10, "error in (no error)"=w307) -> ("error out"=w304:errorcluster)  [unwired: 9 in]
            }
          }
        }
        n93 = for {
          N: 1 -> [_]
          tunnel: [w344] -> w272
          tunnel: w250 -> [w343]
          tunnel: w266 -> [w342]
          tunnel: "TMN DC\\CAP Data Log File Path" -> [w341]
          tunnel: w264 -> [w339]
          tunnel: [w338] -> w228
          tunnel: w260 -> [w326]
          tunnel: w259 -> [w334]
          tunnel: w256 -> [w333]
          tunnel: w253 -> [w332]
          tunnel: [w331] -> w247
          tunnel: w244 -> [w330]
          tunnel: w242 -> [w323]
          tunnel: w237 -> [w328]
          tunnel: w239 -> [w327]
          tunnel: [w326] -> w234
          tunnel: "Sweep CP" -> [w325]
          tunnel: "Init Cycle" -> [w319]
          stop <- w329 stop-if-true
          n94 = case shown="True" w319 {
            tunnel: [w348 w355] -> w324
            tunnel: w323 -> [w348 w354]
            tunnel: "Command" -> [_ w353]
            tunnel: "Post CMd Delay" -> [_ w352]
            tunnel: "Cycle (X1000)" -> [_ w351]
            frame False {
            }
            frame True {
              n95 = call "WS1050_36DUT_Cycle SubVI.vi"("error out"=w354, "Number of Cycle (X1000)"=w351, "Post CMd Delay"=w352, "Command"=w353) -> ("Error Out"=w355:errorcluster, "Cycle Count"=→"Cycle Count":u64)  [unwired: 6 in]
              n96 = local write "STATUS"("Cycling..." ("STATUS")) -> ()
            }
          }
          n97 = while {
            tunnel: w341 -> [w461]
            tunnel: "Test Program" -> [w460]
            tunnel: w327 -> [w459]
            tunnel: "Comment" -> [w458]
            tunnel: "Lot#" -> [w457]
            tunnel: "Wafer#" -> [w456]
            tunnel: w342 -> [w454]
            tunnel: [w455] -> w344
            tunnel: w343 -> [w453]
            tunnel: w339 -> [w451]
            tunnel: [w450] -> w338
            tunnel: [w411] -> w336
            tunnel: [w420] -> w335
            tunnel: w334 -> [w410]
            tunnel: w333 -> [w400]
            tunnel: w332 -> [w399]
            tunnel: [w363] -> w331
            tunnel: w330 -> [w389]
            tunnel: w324 -> [w388]
            tunnel: w328 -> [w383]
            tunnel: w325 -> [w362]
            i -> [w356]
            stop <- w425 stop-if-true
            n98 = case shown="True" w362 {
              tunnel: [w463 w484] -> w398
              tunnel: [w462 w483] -> w397
              tunnel: w388 -> [w466 w482]
              tunnel: w356 -> [w465 w480]
              tunnel: [w464 w481] -> w369
              frame False {
                n99 = case shown="0, 30" w465 {
                  tunnel: w466 -> [w469 w479]
                  tunnel: ["074040" w478] -> w463
                  tunnel: ["0" w477] -> w464
                  tunnel: w465 -> [_ w474]
                  tunnel: [w469 w476] -> w462
                  frame 0, 30 {
                  }
                  frame 1, Default {
                    n100 = call "WS1050 VPI CP Sweep Cmd.vi"("error in (no error)"=w479, "x"=23.0) -> ("error out"=w476:errorcluster, "CP Sweep Cmd"=w470:string[], "Voltage(V)"=w471:string[])  [unwired: 5 in, 2 out]
                    n101 = Subtract(x=w474, y=1) -> (x-y=w472:i32)
                    n102 = Index Array(array=w470, index=w472) -> (element=w478:string)
                    n103 = Index Array(array=w471, index=w472) -> (element=w477:string)
                  }
                }
              }
              frame True {
                n104 = case shown="0, 60" w480 {
                  tunnel: w482 -> [w487 w497]
                  tunnel: ["074040" w495] -> w484
                  tunnel: ["0" w494] -> w481
                  tunnel: w480 -> [_ w490]
                  tunnel: [w487 w492] -> w483
                  frame 0, 60 {
                  }
                  frame 1, Default {
                    n105 = call "WS1050 VPI CP Sweep Cmd.vi"("error in (no error)"=w497, "x"=23.0) -> ("error out"=w492:errorcluster, "Bi_Voltage Out"=w493:string[], "Bi_Cmd Out"=w496:string[])  [unwired: 5 in, 2 out]
                    n106 = Subtract(x=w490, y=1) -> (x-y=w488:i32)
                    n107 = Index Array(array=w496, index=w488) -> (element=w495:string)
                    n108 = Index Array(array=w493, index=w488) -> (element=w494:string)
                  }
                }
              }
            }
            n109 = flat-sequence {
              tunnel: [w501] -> w449
              tunnel: [w510] -> w448
              tunnel: w454 -> [w504]
              tunnel: w453 -> [w522]
              tunnel: [w522] -> w447
              tunnel: [w498] -> w446
              tunnel: [w502] -> w445
              tunnel: w397 -> [w521]
              tunnel: w356 -> [w505]
              tunnel: [w506] -> w424
              tunnel: ["Temperature"] -> w419
              tunnel: w410 -> [w520]
              tunnel: [w520] -> w409
              tunnel: [w519] -> w401
              tunnel: w398 -> [w512]
              tunnel: ["NA" ("Data Out")] -> w392
              tunnel: w383 -> [w515]
              tunnel: [w515] -> w382
              tunnel: [w508] -> w380
              tunnel: w369 -> [w510]
              tunnel: [w510] -> w375
              tunnel: [w512] -> w373
              tunnel: w362 -> [w509]
              tunnel: w362 -> [w507]
              tunnel: [w507] -> w361
              tunnel: w356 -> [w506]
              tunnel: [w645] -> w408
              tunnel: [w644] -> w407
              tunnel: [w643] -> w406
              tunnel: [w642] -> w405
              tunnel: [w641] -> w404
              tunnel: [w640] -> w403
              tunnel: [w628] -> w402
              tunnel: [w639] -> w393
              tunnel: [w638] -> w381
              tunnel: [w635] -> w377
              tunnel: ["WS1050/51"] -> w376
              tunnel: [w637] -> w374
              tunnel: [w636] -> w372
              tunnel: w449 -> [w628]
              tunnel: w448 -> [w645]
              tunnel: w447 -> [w644]
              tunnel: w446 -> [w643]
              tunnel: w445 -> [w642]
              tunnel: w424 -> [w641]
              tunnel: w419 -> [w640]
              tunnel: w409 -> [w633]
              tunnel: w401 -> [w632]
              tunnel: w392 -> [w639]
              tunnel: w382 -> [w638]
              tunnel: w380 -> [w631]
              tunnel: w375 -> [w637]
              tunnel: w373 -> [w636]
              tunnel: ["VPI Name"] -> w366
              tunnel: ["VPI_Cmd"] -> w365
              tunnel: w361 -> [w626]
              tunnel: [w626] -> w360
              tunnel: [w675] -> w444
              tunnel: [w666] -> w443
              tunnel: [w678] -> w442
              tunnel: [w677] -> w441
              tunnel: w408 -> [w676]
              tunnel: [w676] -> w440
              tunnel: w407 -> [w674]
              tunnel: [w674] -> w439
              tunnel: w406 -> [w671]
              tunnel: [w671] -> w438
              tunnel: w405 -> [w670]
              tunnel: [w670] -> w437
              tunnel: w404 -> [w651]
              tunnel: [w651] -> w423
              tunnel: w403 -> [w673]
              tunnel: [w673] -> w418
              tunnel: w402 -> [w672]
              tunnel: [w647] -> w416
              tunnel: [w669] -> w415
              tunnel: [w652] -> w414
              tunnel: [w668] -> w394
              tunnel: w393 -> [w668]
              tunnel: [w667] -> w391
              tunnel: w381 -> [w664]
              tunnel: w377 -> [w663]
              tunnel: w376 -> [w662]
              tunnel: w374 -> [w654]
              tunnel: w372 -> [w655]
              tunnel: [w654] -> w371
              tunnel: w366 -> [w649]
              tunnel: w365 -> [w648]
              tunnel: w360 -> [w646]
              tunnel: [w646] -> w359
              tunnel: [w787] -> w436
              tunnel: [w793] -> w435
              tunnel: [w791] -> w434
              tunnel: [w795] -> w433
              tunnel: [w794] -> w432
              tunnel: [w777] -> w431
              tunnel: [w788] -> w430
              tunnel: [w776] -> w421
              tunnel: [w786] -> w417
              tunnel: [w785] -> w413
              tunnel: [w784] -> w412
              tunnel: "NA" ("Data Out") -> [w783]
              tunnel: [w783] -> w396
              tunnel: [w782] -> w395
              tunnel: [w781] -> w390
              tunnel: ["Freq(Hz)"] -> w379
              tunnel: ["Board#"] -> w378
              tunnel: [w778] -> w370
              tunnel: [w775] -> w367
              tunnel: w371 -> [w778]
              tunnel: w391 -> [w781]
              tunnel: w394 -> [w782]
              tunnel: w414 -> [w785]
              tunnel: w415 -> [w784]
              tunnel: w416 -> [w793]
              tunnel: w418 -> [w786]
              tunnel: w423 -> [w776]
              tunnel: w451 -> [w788]
              tunnel: w437 -> [w789]
              tunnel: w438 -> [w790]
              tunnel: w439 -> [w792]
              tunnel: w440 -> [w777]
              tunnel: w441 -> [w794]
              tunnel: w442 -> [w795]
              tunnel: w443 -> [w775]
              tunnel: w444 -> [w787]
              tunnel: w359 -> [w774]
              tunnel: [w774] -> w358
              tunnel: w436 -> [w838]
              tunnel: w461 -> [w815]
              tunnel: w460 -> [w834]
              tunnel: w459 -> [w836]
              tunnel: w458 -> [w833]
              tunnel: w457 -> [w835]
              tunnel: w456 -> [w832]
              tunnel: [w838] -> w427
              tunnel: [w837] -> w428
              tunnel: w435 -> [w830]
              tunnel: [w830] -> w429
              tunnel: w434 -> [w829]
              tunnel: w433 -> [w828]
              tunnel: w432 -> [w823]
              tunnel: w431 -> [w827]
              tunnel: "File Name" -> [w808]
              tunnel: w430 -> [w826]
              tunnel: [w826] -> w426
              tunnel: [w811] -> w422
              tunnel: w421 -> [w811]
              tunnel: w417 -> [w825]
              tunnel: w413 -> [w824]
              tunnel: w412 -> [w822]
              tunnel: w400 -> [w821]
              tunnel: w389 -> [w820]
              tunnel: w399 -> [w819]
              tunnel: w396 -> [w818]
              tunnel: w395 -> [w817]
              tunnel: w390 -> [w816]
              tunnel: [w813] -> w387
              tunnel: [w804] -> w384
              tunnel: w379 -> [w803]
              tunnel: w378 -> [w801]
              tunnel: w370 -> [w800]
              tunnel: w367 -> [w799]
              tunnel: ["Plot Delta Cmin"] -> w364
              tunnel: w358 -> [w797]
              tunnel: [w796] -> w357
              tunnel: [w859] -> w455
              tunnel: [w860] -> w411
              tunnel: w429 -> [w859]
              tunnel: w428 -> [w853]
              tunnel: w427 -> [w860]
              tunnel: w426 -> [w854]
              tunnel: [w854] -> w450
              tunnel: w422 -> [w850]
              tunnel: [w849] -> w420
              tunnel: [w847] -> w385
              tunnel: w387 -> [w852]
              tunnel: w384 -> [w851]
              tunnel: w364 -> [w846]
              tunnel: w357 -> [w845]
              frame #0 {
                # "Close all drivers, sweep CP"
                n110 = call "WSVCAP SHL Host TL RFFE Write - Multiple DUTs - Common Data.vi"("Data Out"=w512, "error in"=w521, "Log (T)"=FALSE) -> ("error out"=w516:errorcluster)  [unwired: 12 in]
                n111 = for {
                  tunnel: string[] ["0760", "0767", "0768"] -> [w619] mode=indexing
                  tunnel: [w615] -> w517 mode=indexing
                  tunnel: w516 -> [w613]
                  tunnel: [w612] -> w503
                  i -> [w618]
                  n112 = call "Delay.vi"("milliseconds to wait"=u32 10, "error in (no error)"=w613) -> ("error out"=w620:errorcluster)  [unwired: 9 in]
                  n113 = call "WSVCAP SHL Host TL RFFE Read - Multiple DUTs - Common Data.vi"("Data Out"=w619, "error in"=w620, "Log (T)"=FALSE) -> ("RFFE Data In"=w617:string[], "error out"=w612:errorcluster)  [unwired: 11 in]
                  n114 = Index Array(array=w617, index=w618) -> (element=w614:string)
                  n115 = String Subset(string=w614, offset (0)=0) -> (substring=w615:string)  [unwired: 1 in]
                }
                "RB Reg for HD/Cycle" <- w517
                n116 = local read "IDD Brd(uA)"() -> (w499:string)
                n117 = case shown="True" w509 {
                  tunnel: w503 -> [w530 w574]
                  tunnel: [w529 w572] -> w500
                  tunnel: w505 -> [w528 w573]
                  tunnel: w504 -> [w526 w569]
                  tunnel: [w527 w567] -> w502
                  tunnel: [w525 w568] -> w501
                  tunnel: w499 -> [w524 w570]
                  tunnel: [w523 w571] -> w498
                  frame False {
                    n118 = case shown="0, 30" w528 {
                      tunnel: w530 -> [w545 w550 w564]
                      tunnel: [w537 w550 w558] -> w529
                      tunnel: [w536 w548 w551] -> w527
                      tunnel: w526 -> [w535 w549 w556]
                      tunnel: [w534 w549 w553] -> w525
                      tunnel: w524 -> [w532 _ w554]
                      tunnel: [w531 w547 w552] -> w523
                      frame 0, 30 {
                        n119 = call "Delay.vi"("milliseconds to wait"=u32 10, "error in (no error)"=w545) -> ("error out"=w544:errorcluster)  [unwired: 9 in]
                        n120 = call "WSVCAP SHL Host TL RFFE Write - Multiple DUTs - Common Data.vi"("Data Out"="070201000000", "error in"=w544, "Log (T)"=FALSE) -> ("error out"=w538:errorcluster)  [unwired: 12 in]
                        n121 = call "Delay.vi"("milliseconds to wait"=u32 100, "error in (no error)"=w538) -> ("error out"=w540:errorcluster)  [unwired: 9 in]
                        n122 = local read "NOM IDD ON (uA)"() -> (w531:string)
                        n123 = call "Ke2000 Single Reading.vi"("error in (no error)"=w540, "VISA resource name"=w535) -> ("error out"=w541:errorcluster, "VISA resource name out"=w534:refnum<visa-resource-name>, "uA"=w533:string)  [unwired: 5 in, 2 out]
                        n124 = call "Substration.vi"("error in (no error)"=w541, "Input2"=w532, "Input1"=w533) -> ("error out"=w537:errorcluster, "In1 - In2"=w536:string)  [unwired: 7 in]
                      }
                      frame 2, Default {
                        n125 = local read "NOM IDD ON (uA)"() -> (w547:string)
                        n126 = local read "NOM IDD OFF(uA)"() -> (w548:string)
                      }
                      frame 1 {
                        n127 = call "Delay.vi"("milliseconds to wait"=u32 10, "error in (no error)"=w564) -> ("error out"=w563:errorcluster)  [unwired: 9 in]
                        n128 = call "WSVCAP SHL Host TL RFFE Write - Multiple DUTs - Common Data.vi"("Data Out"="0702013B3B3B", "error in"=w563, "Log (T)"=FALSE) -> ("error out"=w557:errorcluster)  [unwired: 12 in]
                        n129 = call "Delay.vi"("milliseconds to wait"=u32 100, "error in (no error)"=w557) -> ("error out"=w560:errorcluster)  [unwired: 9 in]
                        n130 = call "Ke2000 Single Reading.vi"("error in (no error)"=w560, "VISA resource name"=w556) -> ("error out"=w561:errorcluster, "VISA resource name out"=w553:refnum<visa-resource-name>, "uA"=w555:string)  [unwired: 5 in, 2 out]
                        n131 = local read "NOM IDD OFF(uA)"() -> (w551:string)
                        n132 = call "Substration.vi"("error in (no error)"=w561, "Input2"=w554, "Input1"=w555) -> ("error out"=w558:errorcluster, "In1 - In2"=w552:string)  [unwired: 7 in]
                      }
                    }
                  }
                  frame True {
                    n133 = case shown="1" w573 {
                      tunnel: w574 -> [w589 w594 w608]
                      tunnel: [w580 w594 w600] -> w572
                      tunnel: [w585 w593 w599] -> w571
                      tunnel: w570 -> [w576 _ w598]
                      tunnel: w569 -> [w578 w592 w597]
                      tunnel: [w577 w592 w596] -> w568
                      tunnel: [w575 w591 w595] -> w567
                      frame 0, 60 {
                        n134 = call "Delay.vi"("milliseconds to wait"=u32 10, "error in (no error)"=w589) -> ("error out"=w588:errorcluster)  [unwired: 9 in]
                        n135 = call "WSVCAP SHL Host TL RFFE Write - Multiple DUTs - Common Data.vi"("Data Out"="070201000000", "error in"=w588, "Log (T)"=FALSE) -> ("error out"=w579:errorcluster)  [unwired: 12 in]
                        n136 = local read "NOM IDD ON (uA)"() -> (w585:string)
                        n137 = call "Delay.vi"("milliseconds to wait"=u32 100, "error in (no error)"=w579) -> ("error out"=w582:errorcluster)  [unwired: 9 in]
                        n138 = call "Ke2000 Single Reading.vi"("error in (no error)"=w582, "VISA resource name"=w578) -> ("error out"=w583:errorcluster, "VISA resource name out"=w577:refnum<visa-resource-name>, "uA"=w584:string)  [unwired: 5 in, 2 out]
                        n139 = call "Substration.vi"("error in (no error)"=w583, "Input2"=w576, "Input1"=w584) -> ("error out"=w580:errorcluster, "In1 - In2"=w575:string)  [unwired: 7 in]
                      }
                      frame 2, Default {
                        n140 = local read "NOM IDD OFF(uA)"() -> (w591:string)
                        n141 = local read "NOM IDD ON (uA)"() -> (w593:string)
                      }
                      frame 1 {
                        n142 = call "Delay.vi"("milliseconds to wait"=u32 10, "error in (no error)"=w608) -> ("error out"=w607:errorcluster)  [unwired: 9 in]
                        n143 = call "WSVCAP SHL Host TL RFFE Write - Multiple DUTs - Common Data.vi"("Data Out"="0702013B3B3B", "error in"=w607, "Log (T)"=FALSE) -> ("error out"=w601:errorcluster)  [unwired: 12 in]
                        n144 = local read "NOM IDD OFF(uA)"() -> (w595:string)
                        n145 = call "Delay.vi"("milliseconds to wait"=u32 100, "error in (no error)"=w601) -> ("error out"=w603:errorcluster)  [unwired: 9 in]
                        n146 = call "Ke2000 Single Reading.vi"("error in (no error)"=w603, "VISA resource name"=w597) -> ("error out"=w604:errorcluster, "VISA resource name out"=w596:refnum<visa-resource-name>, "uA"=w605:string)  [unwired: 5 in, 2 out]
                        n147 = call "Substration.vi"("error in (no error)"=w604, "Input2"=w598, "Input1"=w605) -> ("error out"=w600:errorcluster, "In1 - In2"=w599:string)  [unwired: 7 in]
                      }
                    }
                  }
                }
                "NOM IDD OFF(uA)" <- w502
                "NOM IDD ON (uA)" <- w498
                n148 = flat-sequence {
                  tunnel: w500 -> [w623]
                  tunnel: [w623] -> w508
                  frame #0 {
                    w624 = "0" ("NOM IDD OFF(uA)")
                    w625 = string[][] []
                    n149 = local write "RB Reg for HD/Cycle"(string[] []) -> ()
                    n150 = local write "NOM IDD ON (uA)"(w624) -> ()
                    n151 = local write "NOM IDD OFF(uA)"(w624) -> ()
                    n152 = local write "VPI C1"(w625) -> ()
                    n153 = local write "VPI C2"(w625) -> ()
                    n154 = local write "VPI C3"(w625) -> ()
                  }
                }
                n155 = local read "Clock Rate (Hz)"() -> (w519:dbl)
              }
              frame #1 {
                n156 = call "WSVCAP SHL Host TL RFFE Configure.vi"("RFFE Slave Address"=w633, "Clock Rate (Hz)"=w632, "error in"=w631) -> ("Actual Rate (Hz)"=w634:dbl, "error out"=w635:errorcluster)  [unwired: 11 in]
                n157 = local write "AR  Measurent(Hz)"(w634) -> ()
              }
              frame #2 {
                n158 = call "WS1050_51 VPI Header CV Curve.vi"("error in (no error)"=w663, "WS1050/51"=w662, "VPI_Cmd"=w648, "VPI Name"=w649) -> ("error out"=w650:errorcluster, "Cmd_3"=w656:string[], "VPI_3"=w659:string[], "VPI Header"=w652:string[], "Cmd_2"=w657:string[], "VPI_2"=w660:string[], "Cmd_1"=w658:string[], "VPI_1"=w661:string[])
                n159 = case shown="True" w664 {
                  tunnel: [w680 w698] -> w653
                  tunnel: [w679 w687] -> w678
                  tunnel: [w679 w685] -> w677
                  tunnel: [_ w699] -> w675
                  tunnel: w672 -> [w682 w706]
                  tunnel: [w682 w706] -> w647
                  tunnel: w658 -> [_ w705]
                  tunnel: w657 -> [_ w702]
                  tunnel: w656 -> [_ w700]
                  tunnel: [w679 w686] -> w669
                  tunnel: w661 -> [_ w704]
                  tunnel: w660 -> [_ w703]
                  tunnel: w659 -> [_ w701]
                  tunnel: ["NA" ("string") w684] -> w667
                  tunnel: w650 -> [w680 w683]
                  tunnel: w654 -> [_ w684]
                  tunnel: w655 -> [_ _]
                  frame False {
                    w679 = string[][] []
                  }
                  frame True {
                    n160 = Array Size(array=w704) -> (size(s)=w688:i32)
                    n161 = for {
                      N: w688 -> [_]
                      tunnel: w705 -> [w769]
                      tunnel: [w753] -> w695
                      tunnel: [w768] -> w697 mode=indexing
                      tunnel: w704 -> [w767]
                      tunnel: w683 -> [w754]
                      tunnel: [w760] -> w690
                      tunnel: w684 -> [w755]
                      i -> [w766]
                      stop <- w753 stop-if-true
                      (unwired) FALSE ("Log (T)")
                      n162 = Index Array(array=w769, index=w766) -> ()  [unwired: 1 out]
                      n163 = Index Array(array=w767, index=w766) -> (element=w758:string)
                      n164 = call <vilib>:"Space Constant.vi"() -> ("String"=w756:string)
                      n165 = Concatenate Strings(w758, w756, w755) -> (w757:string)
                      n166 = call "Delay.vi"("milliseconds to wait"=u32 10, "error in (no error)"=w754) -> ("error out"=w762:errorcluster)  [unwired: 9 in]
                      n167 = local write "STATUS"(w757) -> ()
                      n168 = call "WS1050 AD7747 READ 36 DUT.vi"("error in"=w762, "Log (T)"=FALSE, "DUT Mask Mode (All)"=WSVCAP_SHL_I2C_DUT_Mask_Mode_Enum."C1") -> ("error out"=w764:errorcluster, "AD7747 Values"=w763:string[][])  [unwired: 7 in]
                      n169 = for {
                        tunnel: [w772] -> w768 mode=indexing
                        tunnel: w764 -> [w771]
                        tunnel: [w771] -> w760
                        tunnel: w763 -> [w770] mode=indexing
                        n170 = Index Array(array=w770, index=1) -> (element=w772:string)
                      }
                      n171 = Unbundle By Name(w760) -> ("status"=w753:bool)
                    }
                    n172 = Transpose 2D Array(2D array=w697) -> (transposed array=w687:string[][])
                    "VPI C1" <- w687
                    n173 = Array Size(array=w703) -> (size(s)=w696:i32)
                    n174 = for {
                      N: w696 -> [_]
                      tunnel: w702 -> [w748]
                      tunnel: w695 -> [w746]
                      tunnel: [w745] -> w691
                      tunnel: [w744] -> w694 mode=indexing
                      tunnel: w703 -> [w743]
                      tunnel: w690 -> [w730]
                      tunnel: [w736] -> w689
                      tunnel: w684 -> [w732]
                      i -> [w742]
                      stop <- w745 stop-if-true
                      (unwired) FALSE ("Log (T)")
                      n175 = Index Array(array=w748, index=w742) -> ()  [unwired: 1 out]
                      n176 = Index Array(array=w743, index=w742) -> (element=w734:string)
                      n177 = call <vilib>:"Space Constant.vi"() -> ("String"=w733:string)
                      n178 = Concatenate Strings(w734, w733, w732) -> (w731:string)
                      n179 = call "Delay.vi"("milliseconds to wait"=u32 10, "error in (no error)"=w730) -> ("error out"=w738:errorcluster)  [unwired: 9 in]
                      n180 = call "WS1050 AD7747 READ 36 DUT.vi"("error in"=w738, "Log (T)"=FALSE, "DUT Mask Mode (All)"=WSVCAP_SHL_I2C_DUT_Mask_Mode_Enum."C2") -> ("error out"=w740:errorcluster, "AD7747 Values"=w739:string[][])  [unwired: 7 in]
                      n181 = local write "STATUS"(w731) -> ()
                      n182 = for {
                        tunnel: [w751] -> w744 mode=indexing
                        tunnel: w740 -> [w750]
                        tunnel: [w750] -> w736
                        tunnel: w739 -> [w749] mode=indexing
                        n183 = Index Array(array=w749, index=3) -> (element=w751:string)
                      }
                      n184 = Unbundle By Name(w736) -> ("status"=w747:bool)
                      n185 = Or(x=w747, y=w746) -> (x .or. y?=w745:bool)
                    }
                    n186 = Transpose 2D Array(2D array=w694) -> (transposed array=w686:string[][])
                    "VPI C2" <- w686
                    n187 = Array Size(array=w701) -> (size(s)=w693:i32)
                    n188 = for {
                      N: w693 -> [_]
                      tunnel: w700 -> [w725]
                      tunnel: w691 -> [w723]
                      tunnel: [w722] -> w699
                      tunnel: [w721] -> w692 mode=indexing
                      tunnel: w701 -> [w720]
                      tunnel: w689 -> [w707]
                      tunnel: [w713] -> w698
                      tunnel: w684 -> [w709]
                      i -> [w719]
                      stop <- w722 stop-if-true
                      (unwired) FALSE ("Log (T)")
                      n189 = Index Array(array=w725, index=w719) -> ()  [unwired: 1 out]
                      n190 = Index Array(array=w720, index=w719) -> (element=w711:string)
                      n191 = call <vilib>:"Space Constant.vi"() -> ("String"=w708:string)
                      n192 = call "Delay.vi"("milliseconds to wait"=u32 10, "error in (no error)"=w707) -> ("error out"=w715:errorcluster)  [unwired: 9 in]
                      n193 = Concatenate Strings(w711, w708, w709) -> (w710:string)
                      n194 = call "WS1050 AD7747 READ 36 DUT.vi"("error in"=w715, "Log (T)"=FALSE, "DUT Mask Mode (All)"=WSVCAP_SHL_I2C_DUT_Mask_Mode_Enum."C3") -> ("error out"=w717:errorcluster, "AD7747 Values"=w716:string[][])  [unwired: 7 in]
                      n195 = local write "STATUS"(w710) -> ()
                      n196 = for {
                        tunnel: [w728] -> w721 mode=indexing
                        tunnel: w717 -> [w727]
                        tunnel: [w727] -> w713
                        tunnel: w716 -> [w726] mode=indexing
                        n197 = Index Array(array=w726, index=5) -> (element=w728:string)
                      }
                      n198 = Unbundle By Name(w713) -> ("status"=w724:bool)
                      n199 = Or(x=w724, y=w723) -> (x .or. y?=w722:bool)
                    }
                    n200 = Transpose 2D Array(2D array=w692) -> (transposed array=w685:string[][])
                    "VPI C3" <- w685
                  }
                }
                n201 = call "Delay.vi"("milliseconds to wait"=u32 10, "error in (no error)"=w653) -> ("error out"=w666:errorcluster)  [unwired: 9 in]
              }
              frame #3 {
                n202 = Build Array(w792, w790, w789) -> (w791:string[])
              }
              frame #4 {
                # "Save Data"
                n203 = local write "STATUS"("Saving Data...." ("STATUS")) -> ()
                n204 = Increment(x=w811) -> (x+1=w810:i32)
                n205 = Multiply(x=w810, y=36) -> (x*y=w805:i32)
                n206 = Path To String(path=w815) -> (string=w814:string)
                n207 = Bundle("Test Program"=w834, "Comment"=w833, "Data Out"=w821, "Data Out"=w820, w800, w819, "Data Out"=w818, "Data Out"=w817, "string"=w816, "Freq(Hz)"=w803, "Board#"=w801) -> (w802:T9)  [unwired: 1 in]
                n208 = case shown="True" "Debug" {
                  tunnel: w805 -> [w841 w844]
                  tunnel: [w841 w842] -> w804
                  frame False {
                  }
                  frame True {
                    n209 = Multiply(x=w844, y="No of Rows\nFrom Spread Sheet") -> (x*y=w842:i32)
                  }
                }
                n210 = call "WS1050_36 DUT CV Curve SData Ver1.3.vi"("TMN DC\\CAP Data Log File Path"=w815, "Lot#"=w835, "Wafer#"=w832, "File Name"=w808, "error in"=w799, "TP/Comment"=w802, "Temperature"=w825, "VPI C3"=w823, "VPI C2"=w822, "SN"=w836, "Cap Header"=w824, "HD/Cycles Completed"=w827, "Current"=w829, "VPI C1"=w828) -> ("error out"=w837:errorcluster)  [unwired: 13 in]
                n211 = Concatenate Strings(w814, "\\" ("string"), w808, "_Multi Socket Data.csv" ("string")) -> (w813:string)
                n212 = case shown="False" w797 {
                  tunnel: [30 ("y") 60 ("y")] -> w796
                  frame False {
                  }
                  frame True {
                  }
                }
              }
              frame #5 {
                n213 = case shown="True" w846 {
                  tunnel: w853 -> [w868 w886]
                  tunnel: [w868 w882] -> w848
                  tunnel: w852 -> [_ w878]
                  tunnel: w851 -> [_ w872]
                  frame False {
                  }
                  frame True {
                    n214 = String To Path(string=w878) -> (path=w877:path)
                    n215 = call "Delay.vi"("milliseconds to wait"=u32 50, "error in (no error)"=w886) -> ("error out"=w885:errorcluster)  [unwired: 9 in]
                    n216 = call "36DUT Plot From Spread Sheet Updated.vi"("Col C2"="Col C2", "Col C3"="Col C3", "Plot"="Plot", "No of Rows"=w872, "error in (no error)"=w885, "Col C1"="Col C1", "Bank"="Bank 1", "file path (dialog if empty)"=w877) -> ("error out"=w880:errorcluster, "Delta C_Min Plot"=→"DeltaC Change_1":dbl[][])  [unwired: 2 in]
                    n217 = call "36DUT Plot From Spread Sheet Updated.vi"("Col C2"="Col C2", "Col C3"="Col C3", "Plot"="Plot", "No of Rows"=w872, "error in (no error)"=w880, "Col C1"="Col C1", "Bank"="Bank 2", "file path (dialog if empty)"=w877) -> ("error out"=w881:errorcluster, "Delta C_Min Plot"=→"DeltaC Change_2":dbl[][])  [unwired: 2 in]
                    n218 = call "36DUT Plot From Spread Sheet Updated.vi"("Col C2"="Col C2", "Col C3"="Col C3", "Plot"="Plot", "No of Rows"=w872, "error in (no error)"=w881, "Col C1"="Col C1", "Bank"="Bank 3", "file path (dialog if empty)"=w877) -> ("error out"=w882:errorcluster, "Delta C_Min Plot"=→"DeltaC Change_3":dbl[][])  [unwired: 2 in]
                  }
                }
                n219 = Get Date/Time In Seconds() -> (seconds since 1Jan1904=w855:timestamp)
                n220 = Get Date/Time String(seconds (now)=w855, want seconds? (F)=TRUE) -> (date string=→"date string":string, time string=→"Previous Time":string)  [unwired: 1 in]
                n221 = Greater Or Equal?(x=w850, y=w845) -> (x >= y?=w849:bool)
                n222 = case shown="True" w849 {
                  tunnel: w848 -> [w861 w863]
                  tunnel: [w861 w862] -> w847
                  frame False {
                  }
                  frame True {
                    n223 = call "Delay.vi"("milliseconds to wait"=u32 50, "error in (no error)"=w863) -> ("error out"=w866:errorcluster)  [unwired: 9 in]
                    n224 = call "WSVCAP SHL Host TL RFFE Write - Multiple DUTs - Common Data.vi"("Data Out"="070201000000", "error in"=w866, "Log (T)"=FALSE) -> ("error out"=w862:errorcluster)  [unwired: 12 in]
                  }
                }
                "Loop Completed" <- w850
              }
            }
            n225 = call "Delay.vi"("milliseconds to wait"=u32 10, "error in (no error)"=w385) -> ("error out"=w363:errorcluster)  [unwired: 9 in]
            n226 = Compound Arithmetic op=OR(w411, w420) -> (w425:bool)
          }
          n227 = Unbundle By Name(w331) -> ("status"=w337:bool)
          n228 = Compound Arithmetic op=OR(w337, w336, w335) -> (w329:bool)
        }
        n229 = VISA Write(VISA resource name=w228, write buffer="SOUR:FUNC VOLT;VOLT:MODE FIX;RANG 100;LEV 0.0;:SENS:FUNC \"CURR\";CURR:PROT 60E-3;RANG 100E-3;:OUTP ON", error in (no error)=w247) -> (VISA resource name out=w261:refnum<visa-resource-name>, error out=w246:errorcluster)  [unwired: 1 out]
        n230 = call "E3631A_Voltage Controller updated.vi"("VISA resource name"=w234, "I_VDD(A)"=w222, "Channel Controller"=T7."Voltage 1", "Voltage 1"=0.0, "Voltage 2"=3.3, "error in (no error)"=w247, "I_3.3V (A)"=w222) -> ("VISA resource name out"=w271:refnum<visa-resource-name>, "error out"=w224:errorcluster)  [unwired: 7 in]
        n231 = call "Delay.vi"("milliseconds to wait"=u32 100, "error in (no error)"=w224) -> ("error out"=w245:errorcluster)  [unwired: 9 in]
        n232 = Merge Errors(w245, w246) -> (w262:errorcluster)
      }
      frame True {
      }
    }
    n233 = Wait (ms)(milliseconds to wait=u32 100) -> ()  [unwired: 1 out]
    n234 = Unbundle By Name(w54) -> ("status"=w70:bool)
    n235 = Or(x=w70, y=w62) -> (x .or. y?=w69:bool)
    "STATUS" <- "Idle...." ("STATUS")
  }
  n236 = case shown="True" w22 {
    tunnel: [w903 w906] -> w5
    tunnel: w16 -> [w903 w905]
    frame False {
    }
    frame True {
      n237 = local write "Online"(FALSE ("Online")) -> ()
      n238 = call "WSVCAP SHL Host TL Close.vi"("error in"=w905) -> ("error out"=w906:errorcluster)  [unwired: 14 in]
    }
  }
  n239 = local write "stop"(w10) -> ()
  n240 = VISA Write(VISA resource name=w17, write buffer="SOUR:FUNC VOLT;VOLT:MODE FIX;RANG 100;LEV 0.0;:SENS:FUNC \"CURR\";CURR:PROT 60E-3;RANG 100E-3;:OUTP OFF", error in (no error)=w16) -> (VISA resource name out=w7:refnum<visa-resource-name>, error out=w4:errorcluster)  [unwired: 1 out]
  n241 = Build Array(w9, w8, w7) -> (w6:refnum<visa-resource-name>[])
  n242 = Merge Errors(w5, w4) -> (w3:errorcluster)
  n243 = for {
    tunnel: w6 -> [w909] mode=indexing
    tunnel: w3 -> [w908]
    tunnel: [w907] -> w2
    n244 = VISA Close(VISA resource name=w909, error in (no error)=w908) -> (error out=w907:errorcluster)
  }
  "error out" <- w2
